vi "Process Data PID 0 Set_PD.vi"(0 "Force_peak":sgl, 1 "Force":dbl, 2 "Base force":sgl, 5 "dt IN (s)":dbl=-1.0 format="%.8f", 8 "Num":i32, 10 "PID Set Time(ms)":i32, 11 "output range":cluster{"output high":dbl, "output low":dbl}={"output high"=100.0, "output low"=-100.0} caption="Current Limit" {"output low" format="%.2f"; "output high" format="%.2f"}, 13 "PID gains":T1={"proportional gain (Kc)"=1.0, "integral time (Ti, min)"=0.0, "derivative time (Td, min)"=0.0} caption="force PD Gain" {"derivative time (Td, min)" format="%.7f"; "integral time (Ti, min)" format="%.7f"; "proportional gain (Kc)" format="%.7f"}) -> (14 "current_R":i32 caption="OUTPUT", 17 "Reference force R":dbl, 19 "dt OUT (s)":dbl format="%.8f")   [LabVIEW 2019]
uses:
  <vilib>/addons/control/pid/pid.llb/PID (DBL).vi
  <vilib>/addons/control/pid/NI_PID_pid.lvlib
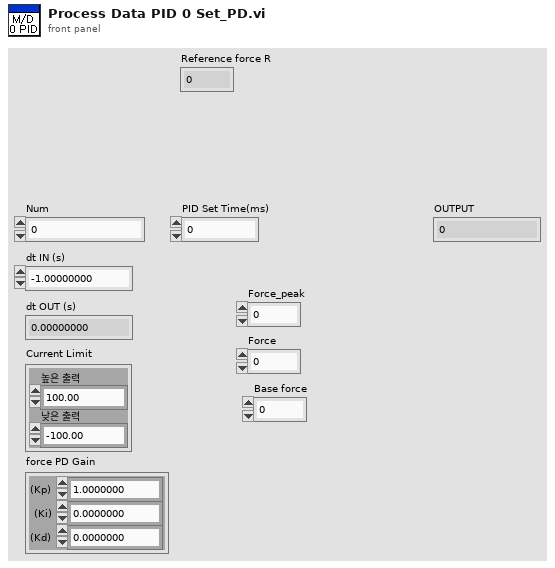
[diagram p1: front panel]
types:
  T1 = cluster{"proportional gain (Kc)":dbl, "integral time (Ti, min)":dbl, "derivative time (Td, min)":dbl}
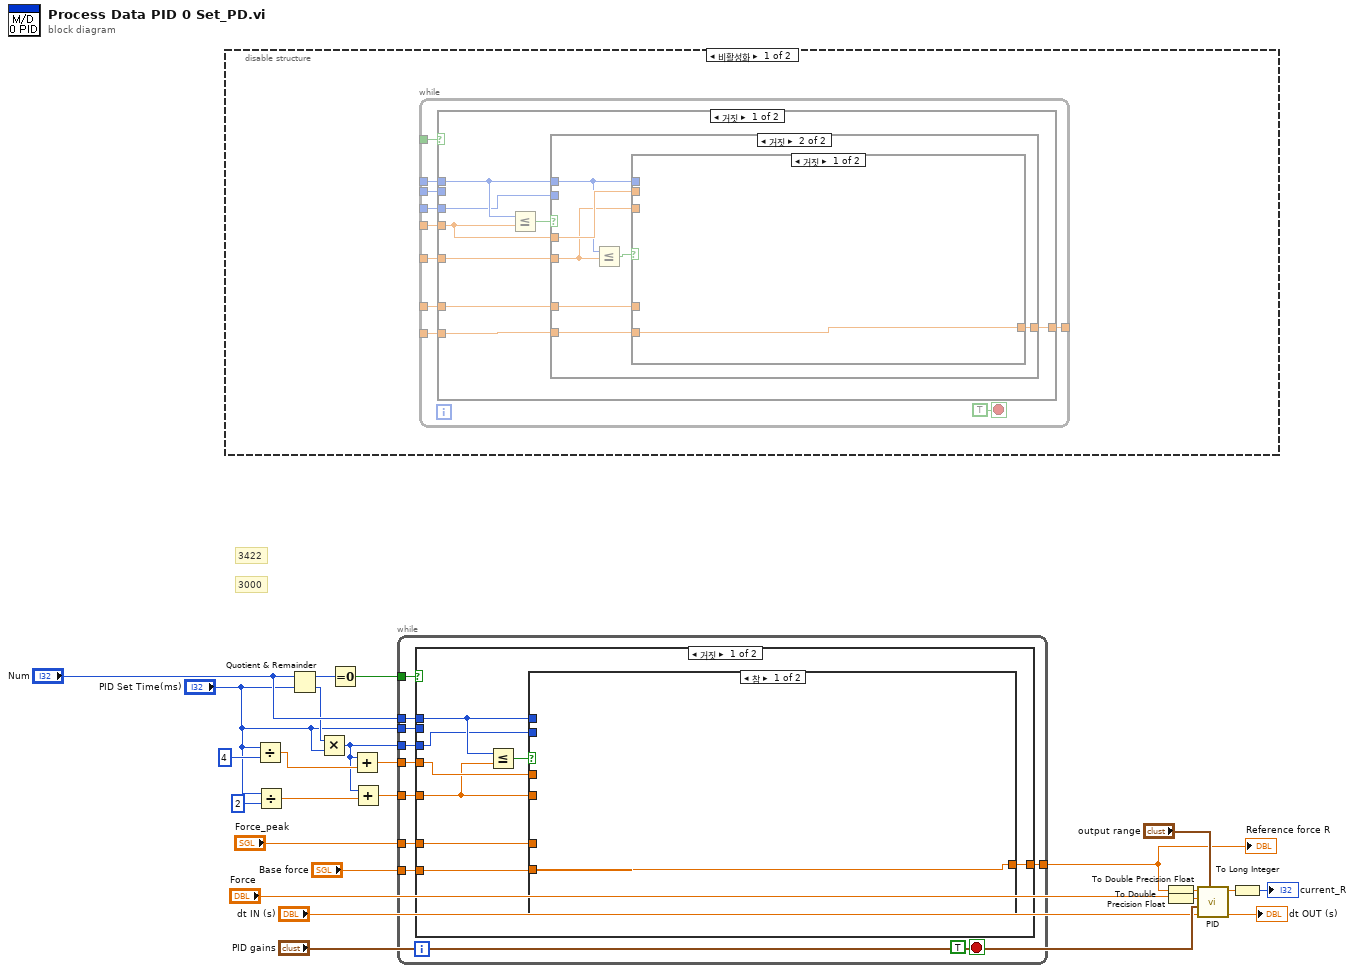
[diagram p0: block diagram]
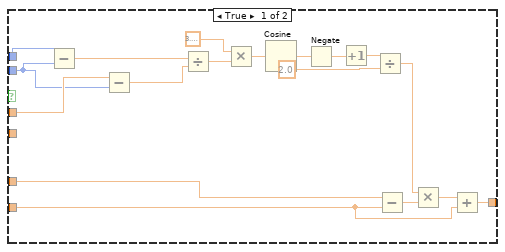
[diagram p2: hidden frame]
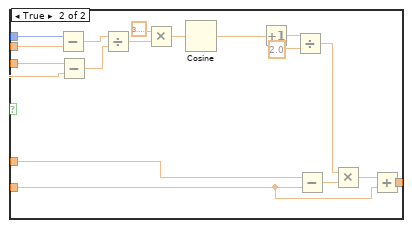
[diagram p3: hidden frame]
diagram:
  # "3000"
  # "3422"
  n1 = disable-structure shown="비활성화" {
    frame Disabled {
      n2 = while {
        tunnel: _ -> [w34]
        tunnel: [w32] -> _
        tunnel: _ -> [w31]
        tunnel: _ -> [w30]
        tunnel: _ -> [w29]
        tunnel: _ -> [w28]
        tunnel: _ -> [w27]
        tunnel: _ -> [w26]
        tunnel: _ -> [w25]
        stop <- TRUE stop-if-true
        n3 = case shown="거짓" w34 {
          tunnel: [w42 w86] -> w32
          tunnel: w31 -> [w41 w86]
          tunnel: w30 -> [w40 _]
          tunnel: w29 -> [w38 _]
          tunnel: w28 -> [_ _]
          tunnel: w27 -> [w37 _]
          tunnel: w26 -> [w36 _]
          tunnel: w25 -> [w35 _]
          frame False {
            n4 = Less Or Equal?(x=w38, y=w36) -> (x <= y?=w39:bool)
            n5 = case shown="거짓" w39 {
              tunnel: w38 -> [w47 w61]
              tunnel: w41 -> [w50 w67]
              tunnel: [w49 w66] -> w42
              tunnel: w40 -> [w48 w65]
              tunnel: w37 -> [w44 _]
              tunnel: w36 -> [w45 w64]
              tunnel: w35 -> [_ w62]
              frame True {
                n6 = Subtract(x=w47, y=w44) -> (x-y=w46:dbl)
                n7 = Subtract(x=w45, y=w44) -> (x-y=w43:dbl)
                n8 = Divide(x=w46, y=w43) -> (x/y=w60:dbl)
                n9 = Multiply(x=3.141592653589793, y=w60) -> (x*y=w58:dbl)
                n10 = Cosine(x=w58) -> (cos(x)=w57:dbl)
                n11 = Negate(x=w57) -> (-x=w56:dbl)
                n12 = Increment(x=w56) -> (x+1=w55:dbl)
                n13 = Divide(x=w55, y=2.0) -> (x/y=w52:dbl)
                n14 = Subtract(x=w48, y=w50) -> (x-y=w53:dbl)
                n15 = Multiply(x=w52, y=w53) -> (x*y=w51:dbl)
                n16 = Add(x=w51, y=w50) -> (x+y=w49:dbl)
              }
              frame False {
                n17 = Less Or Equal?(x=w61, y=w62) -> (x <= y?=w63:bool)
                n18 = case shown="거짓" w63 {
                  tunnel: w67 -> [w68 w85]
                  tunnel: [w68 w84] -> w66
                  tunnel: w65 -> [_ w83]
                  tunnel: w61 -> [_ w82]
                  tunnel: w62 -> [_ w71]
                  tunnel: w64 -> [_ w70]
                  frame False {
                  }
                  frame True {
                    n19 = Subtract(x=w82, y=w70) -> (x-y=w81:dbl)
                    n20 = Subtract(x=w71, y=w70) -> (x-y=w69:dbl)
                    n21 = Divide(x=w81, y=w69) -> (x/y=w80:dbl)
                    n22 = Multiply(x=3.141592653589793, y=w80) -> (x*y=w78:dbl)
                    n23 = Cosine(x=w78) -> (cos(x)=w72:dbl)
                    n24 = Increment(x=w72) -> (x+1=w77:dbl)
                    n25 = Divide(x=w77, y=2.0) -> (x/y=w74:dbl)
                    n26 = Subtract(x=w83, y=w85) -> (x-y=w75:dbl)
                    n27 = Multiply(x=w74, y=w75) -> (x*y=w73:dbl)
                    n28 = Add(x=w73, y=w85) -> (x+y=w84:dbl)
                  }
                }
              }
            }
          }
          frame True {
          }
        }
      }
    }
    frame Enabled {
    }
  }
  n29 = Divide(x="PID Set Time(ms)", y=4) -> (x/y=w7:dbl)
  n30 = Divide(x="PID Set Time(ms)", y=2) -> (x/y=w1:dbl)
  n31 = Quotient & Remainder(x="Num", y="PID Set Time(ms)") -> (x-y*floor(x/y)=w19:i32, floor(x/y)=w9:i32)
  n32 = Multiply(x=w9, y="PID Set Time(ms)") -> (x*y=w5:i32)
  n33 = Equal To 0?(x=w19) -> (x = 0?=w20:bool)
  n34 = Add(x=w5, y=w7) -> (x+y=w6:dbl)
  n35 = Add(x=w5, y=w1) -> (x+y=w4:dbl)
  n36 = while {
    tunnel: w20 -> [w96]
    tunnel: [w94] -> w14
    tunnel: "Base force" -> [w93]
    tunnel: "Force_peak" -> [w92]
    tunnel: "Num" -> [w91]
    tunnel: "PID Set Time(ms)" -> [w90]
    tunnel: w5 -> [w89]
    tunnel: w6 -> [w88]
    tunnel: w4 -> [w87]
    stop <- TRUE stop-if-true
    n37 = case shown="거짓" w96 {
      tunnel: [w104 w107] -> w94
      tunnel: w93 -> [w103 w107]
      tunnel: w92 -> [w102 _]
      tunnel: w91 -> [w100 _]
      tunnel: w90 -> [_ _]
      tunnel: w89 -> [w99 _]
      tunnel: w88 -> [w98 _]
      tunnel: w87 -> [w97 _]
      frame False {
        n38 = Less Or Equal?(x=w100, y=w97) -> (x <= y?=w101:bool)
        n39 = case shown="참" w101 {
          tunnel: w100 -> [_ _]
          tunnel: w103 -> [w105 _]
          tunnel: [w105 w106] -> w104
          tunnel: w102 -> [_ w106]
          tunnel: w99 -> [_ _]
          tunnel: w98 -> [_ _]
          tunnel: w97 -> [_ _]
          frame True {
          }
          frame False {
          }
        }
      }
      frame True {
      }
    }
  }
  "Reference force R" <- w14
  n40 = To Double Precision Float(number=w14) -> (double precision float=w18:dbl)
  n41 = To Double Precision Float(number="Force") -> (double precision float=w17:dbl)
  n42 = call-poly <vilib>:"PID.vi"("output range"="output range", "dt (s)"="dt IN (s)", "PID gains"="PID gains", "process variable"=w17, "setpoint"=w18) -> ("dt out (s)"=→"dt OUT (s)":dbl, "output"=w15:dbl)  [unwired: 5 in]
  n43 = To Long Integer(number=w15) -> (32bit integer=→"current_R":i32)
